vi "RangeI2C_Presets.vi"(0 "Remote IP Address":string="192.168.124.53", 1 "Remote Port":u16=502, 3 "SCL DIO Ch. No.":u16=2, 4 "SDA DIO Ch. No.":u16=3) -> ()   [LabVIEW 2022 SP3]
panel:
  # "Even address values up to 254\n\nInvalid Address Values: 0, 80, 164, 170"
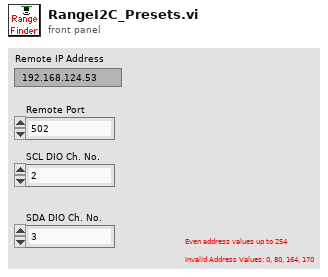
[diagram p1: front panel]
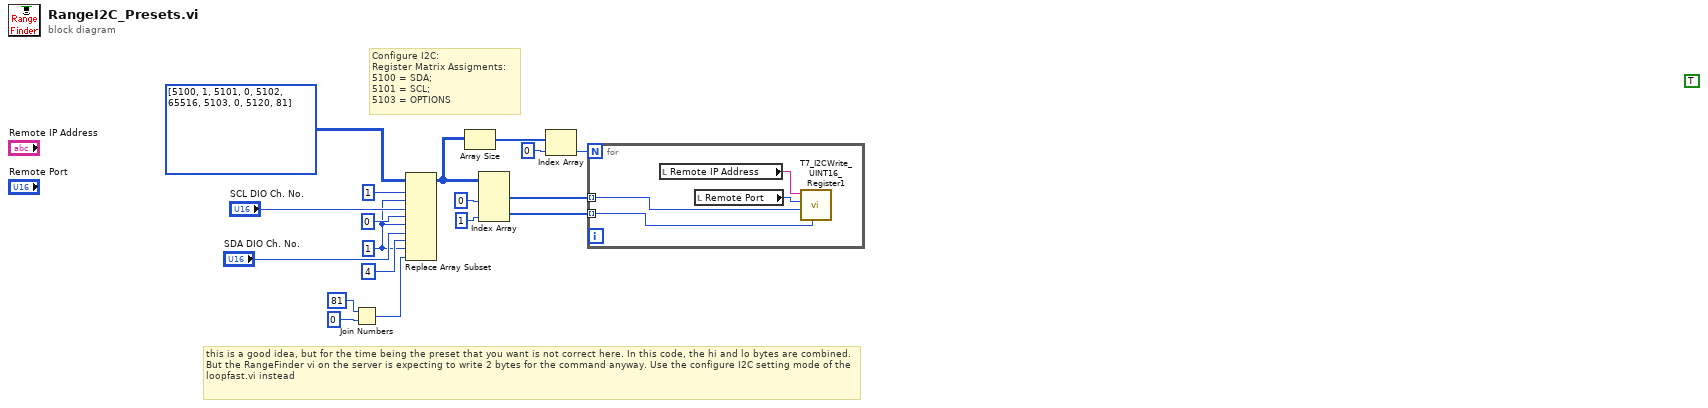
[diagram p0: block diagram]
diagram:
  (unwired) TRUE ("x")
  w1 = 1 ("disabled index (col)")
  # "this is a good idea, but for the time being the preset that you want is not correct here. In this code, the hi and lo bytes are combined. But the RangeFinder vi on the server is expecting to write 2 bytes for the command anyway. Use the configure I2C setting mode of the loopfast.vi instead"
  # "Configure I2C: \nRegister Matrix Assigments:\n5100 = SDA;\n5101 = SCL;\n5103 = OPTIONS"
  n1 = Join Numbers(hi=u16 81, lo=u16 0) -> ((hi.lo)=w2:u32)
  n2 = Replace Array Subset(array=i32[][] [[5100, 1], [5101, 0], [5102, 65516], [5103, 0], [5120, 81]], new element #1="SCL DIO Ch. No.", index (row) #1=1 ("index (row)"), index (col) #1=w1, new element #2="SDA DIO Ch. No.", index (row) #2=0 ("index (row)"), index (col) #2=w1, new element #3=w2, index (row) #3=4 ("index (row)"), index (col) #3=w1) -> (w4:i32[][])
  n3 = Array Size(array=w4) -> (size(s)=w18:i32[])
  n4 = Index Array(array=w4, index (col) #1=0 ("disabled index (col)"), index (col) #2=1 ("index (col)")) -> (element #1=w13:i32[], element #2=w12:i32[])  [unwired: 2 in]
  n5 = Index Array(array=w18, index=0) -> (element=w16:i32)
  n6 = for {
    N: w16 -> [_]
    tunnel: w13 -> [w22] mode=indexing
    tunnel: w12 -> [w21] mode=indexing
    n7 = local read "Remote IP Address"() -> (w20:string)
    n8 = local read "Remote Port"() -> (w19:u16)
    n9 = call "T7_I2CWrite_UINT16_Register1.vi"("Remote IP Address"=w20, "Remote Port"=w19, "Starting Address"=w22, "UINT16 to Write"=w21) -> ()  [unwired: 5 in, 2 out]
  }
